vi "New Title Object.vi"(8 "error in (no error)":errorcluster) -> (0 "error out":errorcluster, 3 "Title out":refnum<class "Title.lvclass">)   [LabVIEW 2017, in "Styles.lvlib" / "Title.lvclass"]
uses:
  Title.lvclass
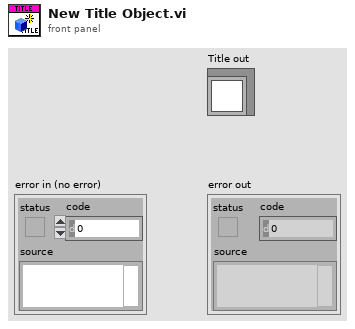
[diagram p1: front panel]
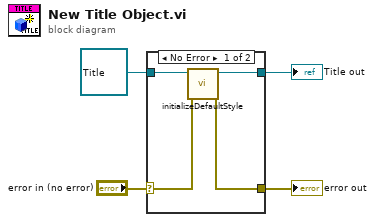
[diagram p0: block diagram]
diagram:
  n1 = case shown="No Error" "error in (no error)" {
    selector: "error in (no error)" -> [w7 w10]
    tunnel: refnum<class "Title.lvclass"> refnum ("Title in") -> [w8 w9]
    tunnel: [w6 w10] -> w2
    tunnel: [w5 w9] -> w1
    frame No Error {
      n2 = call-dynamic "initializeDefaultStyle.vi"("error in (no error)"=w7, "Title in"=w8) -> ("error out"=w6:errorcluster, "Title out"=w5:refnum<class "Title.lvclass">)  [unwired: 8 in]
    }
    frame Error {
    }
  }
  "error out" <- w2
  "Title out" <- w1
